vi "CalculateModulationFreq.vi"(7 "PlanetInfo":T1, 9 "All freq":bool=TRUE, 10 "speed [rpm]":dbl, 11 "Multiple_Frequency":i32) -> (1 "Mesh_Freq":dbl, 2 "char orders out":T2[][](array[typedef]), 3 "char freqs out":T2[][](array[typedef]))   [LabVIEW 2021]
uses:
  Typedefs/Detected peaks.ctl
  Typedefs/PlanetInfo.ctl
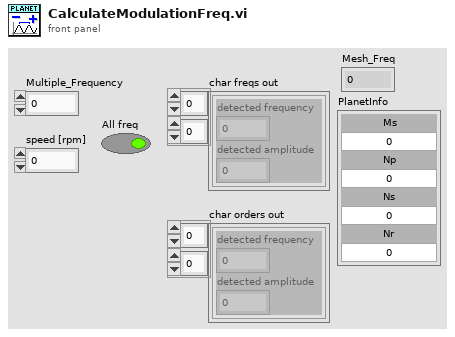
[diagram p1: front panel]
types:
  T1 = typedef "PlanetInfo.ctl" = cluster{"Ms":dbl, "Np":dbl, "Ns":dbl, "Nr":dbl}
  T2 = typedef "Detected peaks.ctl" = cluster{"detected frequency":dbl, "detected amplitude":dbl}
  T3 = cluster{"fm-p":dbl, "fp-p":dbl, "fs":dbl, "fc":dbl, "fp":dbl}
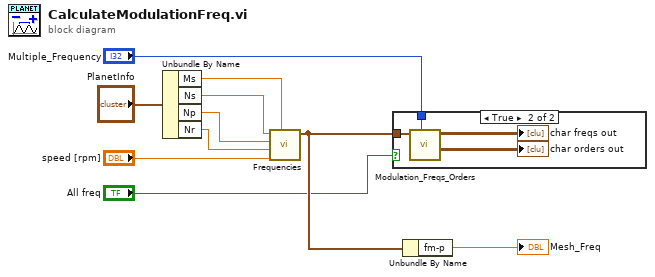
[diagram p0: block diagram]
diagram:
  n1 = Unbundle By Name("PlanetInfo") -> ("Ms"=w4:dbl, "Ns"=w3:dbl, "Np"=w2:dbl, "Nr"=w1:dbl)
  n2 = call "Frequencies.vi"("Mp"=w4, "RPM"="speed [rpm]", "Nr"=w1, "Np"=w2, "Ns"=w3) -> ("char freqs"=w8:T3)  [unwired: 6 in]
  n3 = case shown="True" "All freq" {
    tunnel: "Multiple_Frequency" -> [_ w14]
    tunnel: w8 -> [_ w11]
    frame False {
    }
    frame True {
      n4 = call "Modulation_Freqs_Orders.vi"("Multiple_Frequency"=w14, "char freqs"=w11) -> ("char orders out"=→"char orders out":T2[][], "char freqs out"=→"char freqs out":T2[][])  [unwired: 8 in]
    }
  }
  n5 = Unbundle By Name(w8) -> ("fm-p"=→"Mesh_Freq":dbl)
